vi "JSON Unflatten Configuration.vi"(8 "error in (no error)":errorcluster, 10 "file version":T8, 11 "configuration json":string) -> (0 "error out":errorcluster, 3 "configuration":T1)   [LabVIEW 2017, in "DSF Core.lvlib" / "Configuration Session.lvclass"]
uses:
  Configuration Session.lvclass
  Typedefs/DSF Version Info.ctl
  Typedefs/DSF Engine Framework Configuration.ctl
  Typedefs/DSF Settings Info.ctl
  Typedefs/DSF Engine Plugin Configuration.ctl
  Typedefs/DSF Engine Plugin Thread Configuration.ctl
  Typedefs/DSF Engine Transfer Group Configuration.ctl
  Typedefs/DSF Engine Transfer Configuration.ctl
  Typedefs/DSF Engine Channel Configuration.ctl
  DSF Core.lvlib
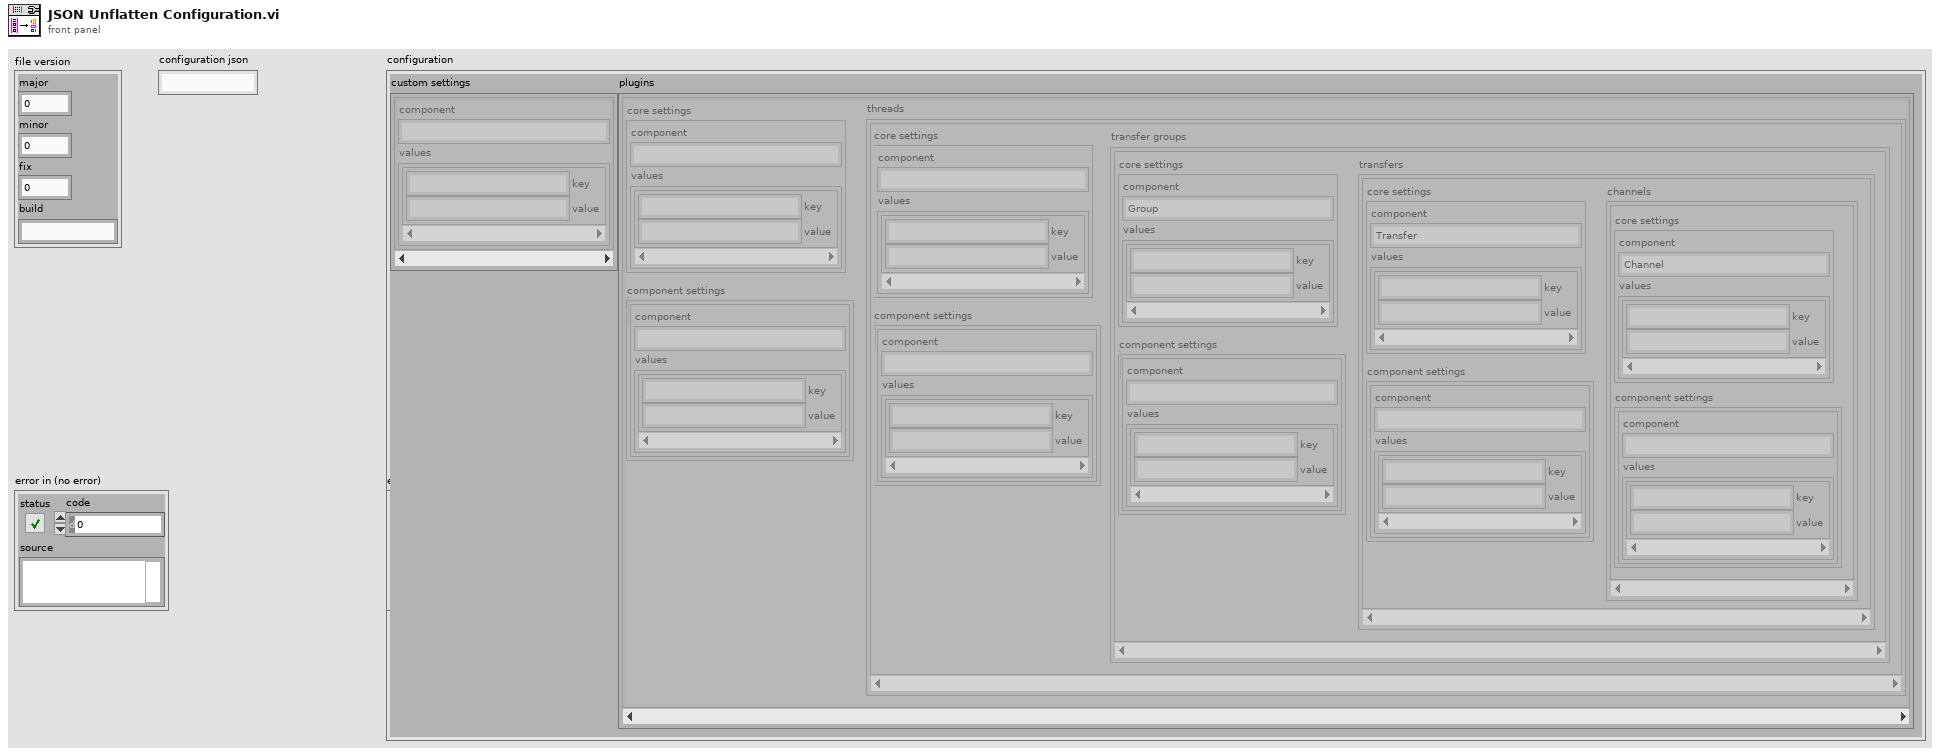
[diagram p1: front panel]
types:
  T1 = typedef "DSF Core.lvlib/DSF Engine Framework Configuration.ctl" = cluster{"custom settings":T2[], "plugins":T3[]}
  T2 = typedef "DSF Core.lvlib/DSF Settings Info.ctl" = cluster{"component":string, "values":cluster{"key":string, "value":string}[]}
  T3 = typedef "DSF Core.lvlib/DSF Engine Plugin Configuration.ctl" = cluster{"core settings":T2, "component settings":T2[], "threads":T4[]}
  T4 = typedef "DSF Core.lvlib/DSF Engine Plugin Thread Configuration.ctl" = cluster{"core settings":T2, "component settings":T2[], "transfer groups":T5[]}
  T5 = typedef "DSF Core.lvlib/DSF Engine Transfer Group Configuration.ctl" = cluster{"core settings":T2, "component settings":T2[], "transfers":T6[]}
  T6 = typedef "DSF Core.lvlib/DSF Engine Transfer Configuration.ctl" = cluster{"core settings":T2, "component settings":T2[], "channels":T7[]}
  T7 = typedef "DSF Core.lvlib/DSF Engine Channel Configuration.ctl" = cluster{"core settings":T2, "component settings":T2[]}
  T8 = typedef "DSF Core.lvlib/DSF Version Info.ctl" = cluster{"major":u32, "minor":u32, "fix":u32, "build":string}
  T9 = cluster{"custom settings":cluster{"component":string, "values":cluster{"key":string, "value":string}[]}[], "plugins":cluster{"core settings":cluster{"component":string, "values":cluster{"key":string, "value":string}[]}, "component settings":cluster{"component":string, "values":cluster{"key":string, "value":string}[]}[], "threads":cluster{"core settings":cluster{"component":string, "values":cluster{"key":string, "value":string}[]}, "component settings":cluster{"component":string, "values":cluster{"key":string, "value":string}[]}[], "transfer groups":cluster{"core settings":cluster{"component":string, "values":cluster{"key":string, "value":string}[]}, "component settings":cluster{"component":string, "values":cluster{"key":string, "value":string}[]}[], "transfers":cluster{"core settings":cluster{"component":string, "values":cluster{"key":string, "value":string}[]}, "component settings":cluster{"component":string, "values":cluster{"key":string, "value":string}[]}[], "channels":cluster{"core settings":cluster{"component":string, "values":cluster{"key":string, "value":string}[]}, "component settings":cluster{"component":string, "values":cluster{"key":string, "value":string}[]}[]}[]}[]}[]}[]}[]}
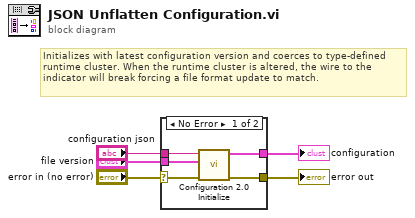
[diagram p0: block diagram]
diagram:
  # "Initializes with latest configuration version and coerces to type-defined runtime cluster. When the runtime cluster is altered, the wire to the indicator will break forcing a file format update to match."
  n1 = case shown="No Error" "error in (no error)" {
    selector: "error in (no error)" -> [w9 w11]
    tunnel: [w10 w11] -> w5
    tunnel: "configuration json" -> [w8 _]
    tunnel: "file version" -> [w7 _]
    tunnel: [w6 _] -> w1
    frame No Error {
      n2 = call "Configuration 2.0 Initialize.vi"("error in (no error)"=w9, "file version"=w7, "configuration json"=w8) -> ("error out"=w10:errorcluster, "configuration 2.0"=w6:T9)  [unwired: 7 in]
    }
    frame Error {
    }
  }
  "error out" <- w5
  "configuration" <- w1
